vi "example_llm_ollama_embedding_unit_test_1.vi"() -> ()   [LabVIEW 2020]
uses:
  src/models/message_vectors/embedding.ctl
  src/models/llm_ollama_embedding/llm_ollama_embedding.lvclass
  src/models/message_text/message_text.lvclass
  D:/lv_llm/labview-llm-libraries/src/models/abstract_message_base/abstract_message_base.lvclass
  src/models/message_text/message.ctl
  src/models/message_vectors/message_vectors.lvclass
panel:
  in  "ollama_url":string="http://localhost:11434/"
  out "property:embedding_data":T1[](array[typedef])
  in  "Text":string[](array[string])=["Hello Pineapple", "LLM embedding is not a", "This is not a Rocket Science"]
  out "error out":errorcluster
  in  "model_name":string(combo)="nomic-embed-text"
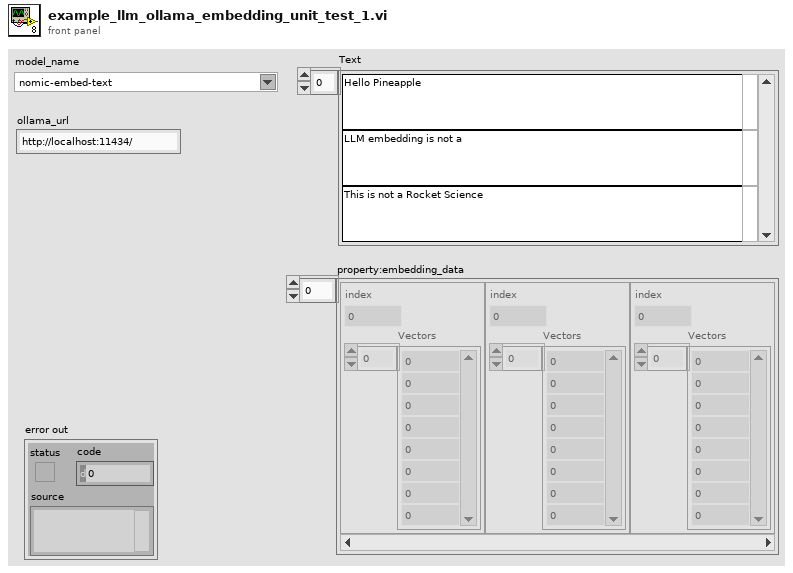
[diagram p1: front panel]
types:
  T1 = typedef "message_vectors.lvclass/embedding.ctl" = cluster{"index":u32, "Vectors":dbl[]}
  T2 = typedef "message_text.lvclass/message.ctl" = cluster{"role":string, "content":string[]}
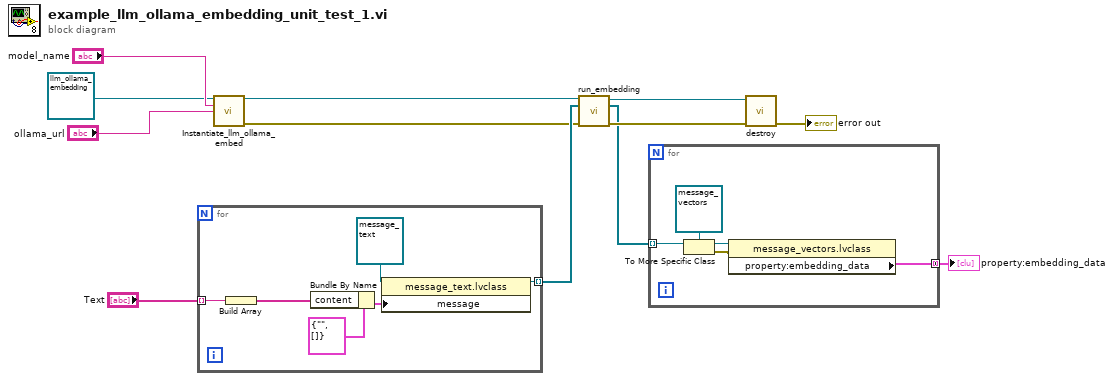
[diagram p0: block diagram]
diagram:
  n1 = for {
    tunnel: "Text" -> [w14] mode=indexing
    tunnel: [w17] -> w8 mode=indexing
    n2 = Build Array(w14) -> (w13:string[])
    n3 = Bundle By Name(cluster=T2 {"role"="", "content"=[]} ("message"), "content"=w13) -> (w15:T2)
    n4 = property class="message_text.lvclass"(reference=refnum<class "message_text.lvclass"> refnum ("message_text.lvclass"), "message"=w15) -> (reference out=w17:refnum<class "message_text.lvclass">)  [unwired: 1 in, 1 out]
  }
  n5 = call "Instantiate_llm_ollama_embed.vi"("llm_ollama_embedding in"=refnum<class "llm_ollama_embedding.lvclass"> refnum ("llm_ollama_embedding.lvclass"), "model_name"="model_name", "ollama_url"="ollama_url") -> ("llm_ollama_embedding out"=w12:refnum<class "llm_ollama_embedding.lvclass">, "error out"=w6:errorcluster)  [unwired: 11 in]
  n6 = call-dynamic "run_embedding.vi"("llm_ollama_embedding in"=w12, "data"=w8, "error in (no error)"=w6) -> ("llm_ollama_embedding out"=w11:refnum<class "llm_ollama_embedding.lvclass">, "embedding response"=w4:refnum<class "message_vectors.lvclass">[], "error out"=w10:errorcluster)  [unwired: 10 in]
  n7 = for {
    tunnel: [w23] -> w3 mode=concatenating
    tunnel: w4 -> [w19] mode=indexing
    n8 = To More Specific Class(target class=refnum<class "message_vectors.lvclass"> refnum ("message_vectors.lvclass"), reference=w19) -> (specific class reference=w20:refnum<class "message_vectors.lvclass">, error out=w22:errorcluster)  [unwired: 1 in]
    n9 = property class="message_vectors.lvclass"(reference=w20, error in=w22) -> ("property:embedding_data"=w23:T1[])  [unwired: 2 out]
  }
  "property:embedding_data" <- w3
  n10 = call-dynamic "destroy.vi"("error in (no error)"=w10, "llm_ollama_embedding in"=w11) -> ("error out"=→"error out":errorcluster)  [unwired: 8 in, 1 out]
